vi "LINC Command Record.vi"(8 "error in (no error)":errorcluster, 10 "command text":string, 11 "LINC session":refnum<class "LINC.lvclass">) -> (0 "error out":errorcluster, 3 "dup LINC session":refnum<class "LINC.lvclass">)   [LabVIEW 2018, in "STEPkgDriver_LINC.lvlib" / "LINC.lvclass"]
uses:
  LINC.lvclass
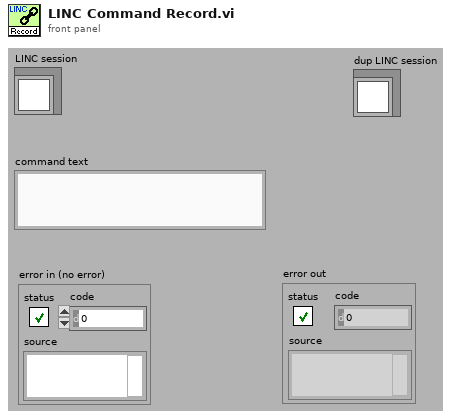
[diagram p1: front panel]
types:
  T1 = enum16{"open", "replace", "create", "open or create", "replace or create", "replace or create with confirmation"}
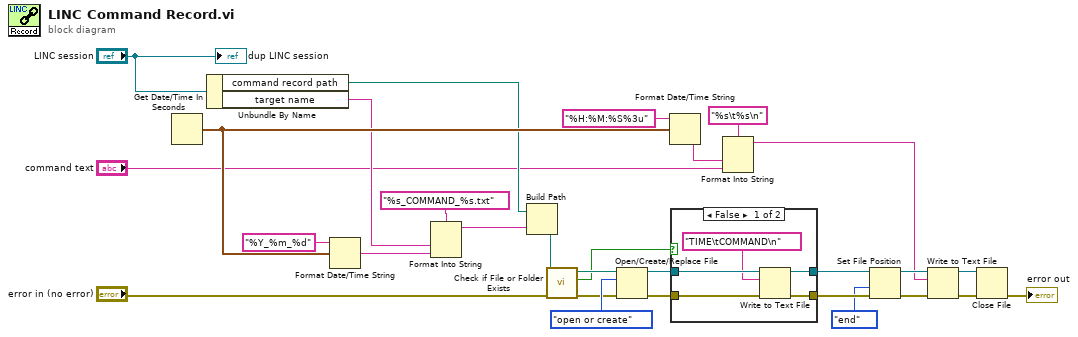
[diagram p0: block diagram]
diagram:
  n1 = Get Date/Time In Seconds() -> (seconds since 1Jan1904=w6:timestamp)
  n2 = Unbundle By Name("LINC session") -> ("command record path"=w4:path, "target name"=w3:string)
  n3 = Format Date/Time String(time format string (%c)="%Y_%m_%d", seconds (now)=w6) -> (date/time string=w8:string)  [unwired: 1 in]
  n4 = Format Into String(format string="%s_COMMAND_%s.txt", w3, w8) -> (resulting string=w7:string)  [unwired: 2 in, 1 out]
  n5 = Build Path(base path=w4, name or relative path=w7) -> (appended path=w17:path)
  n6 = call <vilib>:"Check if File or Folder Exists.vi"("error in (no error)"="error in (no error)", "path"=w17) -> ("error out"=w18:errorcluster, "file or folder exists?"=w15:bool, "dup path"=w16:path)  [unwired: 7 in]
  n7 = Open/Create/Replace File(file path (use dialog)=w16, error in=w18, operation (0:open)=T1."open or create") -> (refnum out=w27:refnum<file>, error out=w26:errorcluster)  [unwired: 3 in, 1 out]
  n8 = Format Date/Time String(time format string (%c)="%H:%M:%S%3u", seconds (now)=w6) -> (date/time string=w11:string)  [unwired: 1 in]
  n9 = case shown="False" w15 {
    tunnel: w26 -> [w34 w36]
    tunnel: [w32 w36] -> w25
    tunnel: w27 -> [w33 w35]
    tunnel: [w31 w35] -> w24
    frame False {
      n10 = Write to Text File(file (use dialog)=w33, text="TIME\tCOMMAND\n", error in=w34) -> (refnum out=w31:refnum<file>, error out=w32:errorcluster)  [unwired: 1 in, 1 out]
    }
    frame True {
    }
  }
  n11 = Format Into String(format string="%s\t%s\n", w11, "command text") -> (resulting string=w12:string)  [unwired: 2 in, 1 out]
  n12 = Set File Position(refnum=w24, from (0:start)=enum16{"start", "end", "current"}."end", error in=w25) -> (refnum out=w21:refnum<file>, error out=w22:errorcluster)  [unwired: 1 in]
  n13 = Write to Text File(file (use dialog)=w21, text=w12, error in=w22) -> (refnum out=w19:refnum<file>, error out=w20:errorcluster)  [unwired: 1 in, 1 out]
  n14 = Close File(refnum=w19, error in=w20) -> (error out=→"error out":errorcluster)  [unwired: 1 out]
  "dup LINC session" <- "LINC session"
